vi "Instructor Write Client.vi"() -> ()   [LabVIEW 2017]
uses:
  <vilib>/OPCUA/controls/Write Status.ctl
  <vilib>/OPCUA/controls/NodeId.ctl
  <vilib>/OPCUA/client/Multiple Write Double Array.vi
  <vilib>/OPCUA/client/Multiple Write Bool Array.vi
  <vilib>/OPCUA/NI OPC UA Client.lvlib
panel:
  in  "Node Status 2":T1 items=["Good"=0, "Uncertain_InitialValue"=1083310080, "Uncertain_LastUsableValue"=1083179008, "Uncertain_SensorNotAccurate"=1083375616, "Uncertain_EngineeringUnitsExceeded"=1083441152, "Bad_NoCommunication"=2150694912, "Bad_NotReadable"=2151284736, "Bad_NotWritable"=2151350272, "Bad_OutOfRange"=2151415808, "Bad_WaitingForInitialData"=2150760448]
  in  "Time Stamp 2":timestamp
  in  "Node Status":T1 items=["Good"=0, "Uncertain_InitialValue"=1083310080, "Uncertain_LastUsableValue"=1083179008, "Uncertain_SensorNotAccurate"=1083375616, "Uncertain_EngineeringUnitsExceeded"=1083441152, "Bad_NoCommunication"=2150694912, "Bad_NotReadable"=2151284736, "Bad_NotWritable"=2151350272, "Bad_OutOfRange"=2151415808, "Bad_WaitingForInitialData"=2150760448]
  in  "Time Stamp":timestamp
  in  "Stop Broadcasting":bool
  in  "Time Stamp":timestamp
  in  "Node Status":T1 items=["Good"=0, "Uncertain_InitialValue"=1083310080, "Uncertain_LastUsableValue"=1083179008, "Uncertain_SensorNotAccurate"=1083375616, "Uncertain_EngineeringUnitsExceeded"=1083441152, "Bad_NoCommunication"=2150694912, "Bad_NotReadable"=2151284736, "Bad_NotWritable"=2151350272, "Bad_OutOfRange"=2151415808, "Bad_WaitingForInitialData"=2150760448]
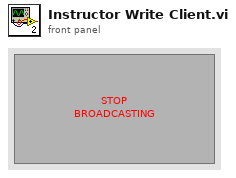
[diagram p1: front panel]
types:
  T1 = typedef "Write Status.ctl" = u32
  T2 = cluster{"message mode":enum16{"None", "Sign", "Sign and Encrypt"}, "security":enum16{"Basic256", "Basic128Rsa15"}}
  T3 = typedef "OPC UA Client Refnum.ctl" = refnum<k21>
  T4 = typedef "NodeId.ctl" = string
  T5 = cluster{"node ID":T4, "value":bool[], "timestamp (current time)":timestamp, "node status":T1}
  T6 = cluster{"node ID":T4, "value":dbl[], "timestamp (current time)":timestamp, "node status":T1}
  T7 = cluster{"node ID":T4, "value":dbl[], "timestamp (current time)":timestamp, "node status":T1}[]
  T8 = cluster{"node ID":T4, "value":bool[], "timestamp (current time)":timestamp, "node status":T1}[]
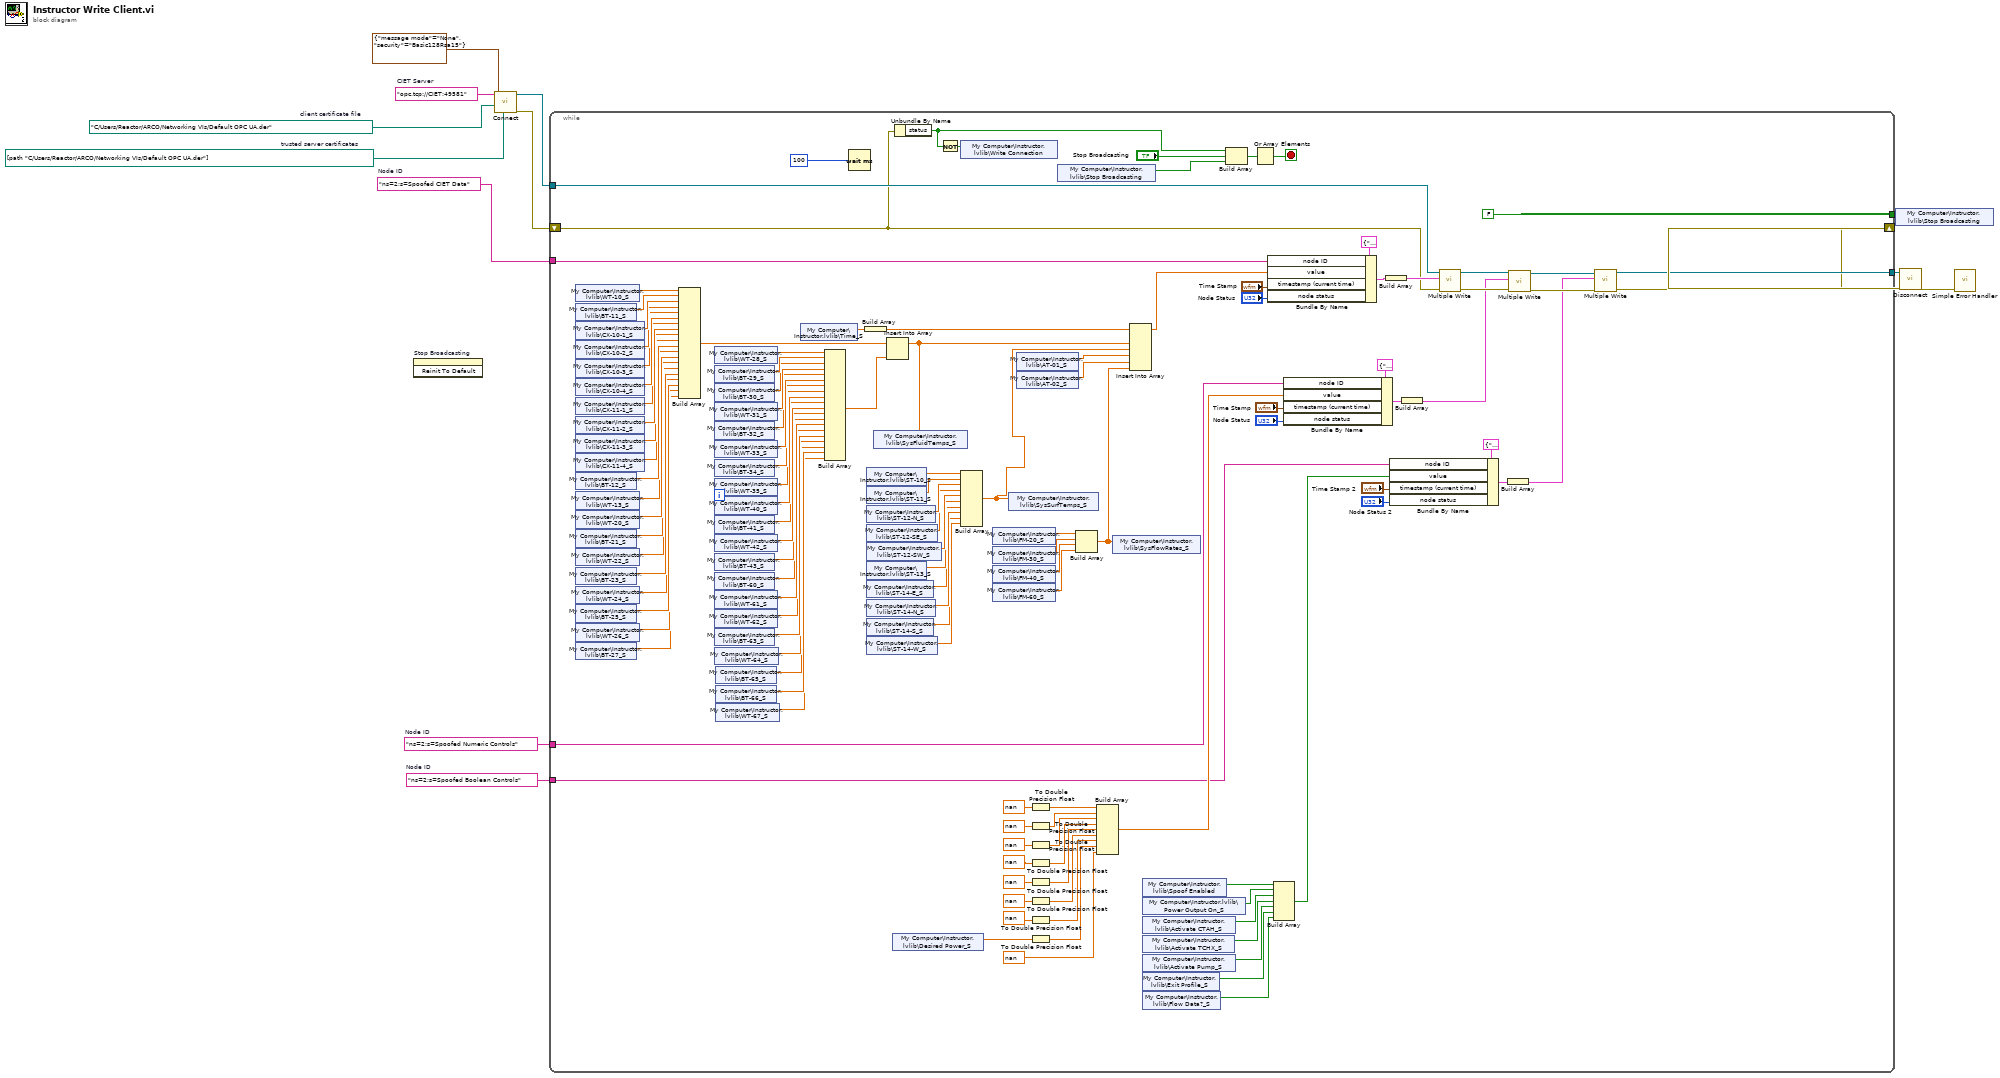
[diagram p0: block diagram]
diagram:
  w1 = "ns=2;s=Spoofed Boolean Controls"  # Node ID
  w3 = "ns=2;s=Spoofed Numeric Controls"  # Node ID
  w8 = path[] [path "C:/Users/Reactor/ARCO/Networking VIs/Default OPC UA.der"]  # trusted server certificates
  w9 = path "C:/Users/Reactor/ARCO/Networking VIs/Default OPC UA.der"  # client certificate file
  w10 = "ns=2;s=Spoofed CIET Data"  # Node ID
  w12 = "opc.tcp://CIET:49581"  # CIET Server
  n1 = invoke on="Stop Broadcasting" class="Bool (strict)" method="Reinit To Default"() -> ()  [unwired: 3 in, 3 out]
  n2 = call <vilib>:"Connect.vi"("trusted server certificates"=w8, "client certificate file"=w9, "security policy"=T2 {"message mode"=enum."None", "security"=enum."Basic128Rsa15"}, "server endpoint URL"=w12) -> ("error out"=w5:errorcluster, "OPC UA client refnum out"=w11:T3)  [unwired: 5 in, 1 out]
  n3 = while {
    tunnel: w10 -> [w136]
    tunnel: w11 -> [w135]
    tunnel: [FALSE] -> w6
    shift-right: [w24] -> w4
    shift-left: w5 -> [w58]
    tunnel: w3 -> [w52]
    tunnel: [w25] -> w2
    tunnel: w1 -> [w23]
    stop <- w64 stop-if-true
    n4 = shared-variable "My Computer\\Instructor.lvlib\\WT-10_S"() -> (w129:sgl)  [unwired: 1 in, 1 out]
    n5 = shared-variable "My Computer\\Instructor.lvlib\\BT-11_S"() -> (w128:sgl)  [unwired: 1 in, 1 out]
    n6 = shared-variable "My Computer\\Instructor.lvlib\\CX-10-1_S"() -> (w127:sgl)  [unwired: 1 in, 1 out]
    n7 = shared-variable "My Computer\\Instructor.lvlib\\CX-10-2_S"() -> (w126:sgl)  [unwired: 1 in, 1 out]
    n8 = shared-variable "My Computer\\Instructor.lvlib\\CX-10-3_S"() -> (w125:sgl)  [unwired: 1 in, 1 out]
    n9 = shared-variable "My Computer\\Instructor.lvlib\\CX-10-4_S"() -> (w124:sgl)  [unwired: 1 in, 1 out]
    n10 = shared-variable "My Computer\\Instructor.lvlib\\CX-11-1_S"() -> (w123:sgl)  [unwired: 1 in, 1 out]
    n11 = shared-variable "My Computer\\Instructor.lvlib\\CX-11-2_S"() -> (w122:sgl)  [unwired: 1 in, 1 out]
    n12 = shared-variable "My Computer\\Instructor.lvlib\\CX-11-3_S"() -> (w121:sgl)  [unwired: 1 in, 1 out]
    n13 = shared-variable "My Computer\\Instructor.lvlib\\CX-11-4_S"() -> (w120:sgl)  [unwired: 1 in, 1 out]
    n14 = shared-variable "My Computer\\Instructor.lvlib\\BT-12_S"() -> (w119:sgl)  [unwired: 1 in, 1 out]
    n15 = shared-variable "My Computer\\Instructor.lvlib\\WT-13_S"() -> (w118:sgl)  [unwired: 1 in, 1 out]
    n16 = shared-variable "My Computer\\Instructor.lvlib\\WT-20_S"() -> (w117:sgl)  [unwired: 1 in, 1 out]
    n17 = shared-variable "My Computer\\Instructor.lvlib\\BT-21_S"() -> (w116:sgl)  [unwired: 1 in, 1 out]
    n18 = shared-variable "My Computer\\Instructor.lvlib\\WT-22_S"() -> (w115:sgl)  [unwired: 1 in, 1 out]
    n19 = shared-variable "My Computer\\Instructor.lvlib\\BT-23_S"() -> (w114:sgl)  [unwired: 1 in, 1 out]
    n20 = shared-variable "My Computer\\Instructor.lvlib\\WT-24_S"() -> (w113:sgl)  [unwired: 1 in, 1 out]
    n21 = shared-variable "My Computer\\Instructor.lvlib\\BT-25_S"() -> (w112:sgl)  [unwired: 1 in, 1 out]
    n22 = shared-variable "My Computer\\Instructor.lvlib\\WT-26_S"() -> (w111:sgl)  [unwired: 1 in, 1 out]
    n23 = shared-variable "My Computer\\Instructor.lvlib\\BT-27_S"() -> (w110:sgl)  [unwired: 1 in, 1 out]
    n24 = Build Array(w129, w128, w127, w126, w125, w124, w123, w122, w121, w120, w119, w118, w117, w116, w115, w114, w113, w112, w111, w110) -> (w88:sgl[])
    n25 = shared-variable "My Computer\\Instructor.lvlib\\WT-28_S"() -> (w109:sgl)  [unwired: 1 in, 1 out]
    n26 = shared-variable "My Computer\\Instructor.lvlib\\BT-29_S"() -> (w108:sgl)  [unwired: 1 in, 1 out]
    n27 = shared-variable "My Computer\\Instructor.lvlib\\BT-30_S"() -> (w107:sgl)  [unwired: 1 in, 1 out]
    n28 = shared-variable "My Computer\\Instructor.lvlib\\WT-31_S"() -> (w106:sgl)  [unwired: 1 in, 1 out]
    n29 = shared-variable "My Computer\\Instructor.lvlib\\BT-32_S"() -> (w105:sgl)  [unwired: 1 in, 1 out]
    n30 = shared-variable "My Computer\\Instructor.lvlib\\WT-33_S"() -> (w104:sgl)  [unwired: 1 in, 1 out]
    n31 = shared-variable "My Computer\\Instructor.lvlib\\BT-34_S"() -> (w103:sgl)  [unwired: 1 in, 1 out]
    n32 = shared-variable "My Computer\\Instructor.lvlib\\WT-35_S"() -> (w102:sgl)  [unwired: 1 in, 1 out]
    n33 = shared-variable "My Computer\\Instructor.lvlib\\WT-40_S"() -> (w101:sgl)  [unwired: 1 in, 1 out]
    n34 = shared-variable "My Computer\\Instructor.lvlib\\BT-41_S"() -> (w100:sgl)  [unwired: 1 in, 1 out]
    n35 = shared-variable "My Computer\\Instructor.lvlib\\WT-42_S"() -> (w99:sgl)  [unwired: 1 in, 1 out]
    n36 = shared-variable "My Computer\\Instructor.lvlib\\BT-43_S"() -> (w98:sgl)  [unwired: 1 in, 1 out]
    n37 = shared-variable "My Computer\\Instructor.lvlib\\BT-60_S"() -> (w97:sgl)  [unwired: 1 in, 1 out]
    n38 = shared-variable "My Computer\\Instructor.lvlib\\WT-61_S"() -> (w96:sgl)  [unwired: 1 in, 1 out]
    n39 = shared-variable "My Computer\\Instructor.lvlib\\WT-62_S"() -> (w95:sgl)  [unwired: 1 in, 1 out]
    n40 = shared-variable "My Computer\\Instructor.lvlib\\BT-63_S"() -> (w94:sgl)  [unwired: 1 in, 1 out]
    n41 = shared-variable "My Computer\\Instructor.lvlib\\WT-64_S"() -> (w93:sgl)  [unwired: 1 in, 1 out]
    n42 = shared-variable "My Computer\\Instructor.lvlib\\BT-65_S"() -> (w92:sgl)  [unwired: 1 in, 1 out]
    n43 = shared-variable "My Computer\\Instructor.lvlib\\BT-66_S"() -> (w91:sgl)  [unwired: 1 in, 1 out]
    n44 = shared-variable "My Computer\\Instructor.lvlib\\WT-67_S"() -> (w90:sgl)  [unwired: 1 in, 1 out]
    n45 = shared-variable "My Computer\\Instructor.lvlib\\Time_S"() -> (w77:sgl)  [unwired: 1 in, 1 out]
    n46 = Build Array(w109, w108, w107, w106, w105, w104, w103, w102, w101, w100, w99, w98, w97, w96, w95, w94, w93, w92, w91, w90) -> (w89:sgl[])
    n47 = Wait (ms)(milliseconds to wait=u32 100) -> ()  [unwired: 1 out]
    n48 = Build Array(w77) -> (w68:sgl[])
    n49 = shared-variable "My Computer\\Instructor.lvlib\\ST-10_S"() -> (w87:sgl)  [unwired: 1 in, 1 out]
    n50 = shared-variable "My Computer\\Instructor.lvlib\\ST-11_S"() -> (w86:sgl)  [unwired: 1 in, 1 out]
    n51 = shared-variable "My Computer\\Instructor.lvlib\\ST-12-N_S"() -> (w85:sgl)  [unwired: 1 in, 1 out]
    n52 = shared-variable "My Computer\\Instructor.lvlib\\ST-12-SE_S"() -> (w84:sgl)  [unwired: 1 in, 1 out]
    n53 = shared-variable "My Computer\\Instructor.lvlib\\ST-12-SW_S"() -> (w83:sgl)  [unwired: 1 in, 1 out]
    n54 = shared-variable "My Computer\\Instructor.lvlib\\ST-13_S"() -> (w82:sgl)  [unwired: 1 in, 1 out]
    n55 = shared-variable "My Computer\\Instructor.lvlib\\ST-14-E_S"() -> (w81:sgl)  [unwired: 1 in, 1 out]
    n56 = shared-variable "My Computer\\Instructor.lvlib\\ST-14-N_S"() -> (w80:sgl)  [unwired: 1 in, 1 out]
    n57 = shared-variable "My Computer\\Instructor.lvlib\\ST-14-S_S"() -> (w79:sgl)  [unwired: 1 in, 1 out]
    n58 = shared-variable "My Computer\\Instructor.lvlib\\ST-14-W_S"() -> (w78:sgl)  [unwired: 1 in, 1 out]
    n59 = Insert Into Array(array=w88, new element=w89) -> (w76:sgl[])  [unwired: 1 in]
    n60 = shared-variable "My Computer\\Instructor.lvlib\\SysFluidTemps_S"(w76) -> ()  [unwired: 1 in, 1 out]
    n61 = shared-variable "My Computer\\Instructor.lvlib\\Desired Power_S"() -> (w45:sgl)  [unwired: 1 in, 1 out]
    n62 = Unbundle By Name(w58) -> ("status"=w60:bool)
    n63 = Not(x=w60) -> (.not. x?=w59:bool)
    n64 = shared-variable "My Computer\\Instructor.lvlib\\Write Connection"(w59) -> ()  [unwired: 1 in, 1 out]
    n65 = Build Array(w87, w86, w85, w84, w83, w82, w81, w80, w79, w78) -> (w67:sgl[])
    n66 = shared-variable "My Computer\\Instructor.lvlib\\FM-20_S"() -> (w73:sgl)  [unwired: 1 in, 1 out]
    n67 = shared-variable "My Computer\\Instructor.lvlib\\FM-30_S"() -> (w72:sgl)  [unwired: 1 in, 1 out]
    n68 = shared-variable "My Computer\\Instructor.lvlib\\FM-40_S"() -> (w71:sgl)  [unwired: 1 in, 1 out]
    n69 = shared-variable "My Computer\\Instructor.lvlib\\FM-60_S"() -> (w70:sgl)  [unwired: 1 in, 1 out]
    n70 = shared-variable "My Computer\\Instructor.lvlib\\SysSurfTemps_S"(w67) -> ()  [unwired: 1 in, 1 out]
    n71 = shared-variable "My Computer\\Instructor.lvlib\\AT-01_S"() -> (w75:sgl)  [unwired: 1 in, 1 out]
    n72 = shared-variable "My Computer\\Instructor.lvlib\\AT-02_S"() -> (w74:sgl)  [unwired: 1 in, 1 out]
    n73 = To Double Precision Float(number=nan) -> (double precision float=w49:dbl)
    n74 = To Double Precision Float(number=nan) -> (double precision float=w48:dbl)
    n75 = To Double Precision Float(number=nan) -> (double precision float=w47:dbl)
    n76 = To Double Precision Float(number=nan) -> (double precision float=w46:dbl)
    n77 = To Double Precision Float(number=nan) -> (double precision float=w44:dbl)
    n78 = To Double Precision Float(number=nan) -> (double precision float=w43:dbl)
    n79 = To Double Precision Float(number=nan) -> (double precision float=w42:dbl)
    n80 = To Double Precision Float(number=w45) -> (double precision float=w41:dbl)
    n81 = shared-variable "My Computer\\Instructor.lvlib\\Stop Broadcasting"() -> (w62:bool)  [unwired: 1 in, 1 out]
    n82 = Build Array(w73, w72, w71, w70) -> (w69:sgl[])
    n83 = Build Array(w49, w48, w47, w46, w44, w43, w42, w41, nan ("number")) -> (w40:dbl[])
    n84 = shared-variable "My Computer\\Instructor.lvlib\\SysFlowRates_S"(w69) -> ()  [unwired: 1 in, 1 out]
    n85 = Insert Into Array(array=w68, new element #1=w76, new element #2=w67, new element #3=w75, new element #4=w74, new element #5=w69) -> (w66:sgl[])  [unwired: 1 in]
    n86 = shared-variable "My Computer\\Instructor.lvlib\\Spoof Enabled"() -> (w21:bool)  [unwired: 1 in, 1 out]
    n87 = shared-variable "My Computer\\Instructor.lvlib\\Power Output On_S"() -> (w20:bool)  [unwired: 1 in, 1 out]
    n88 = shared-variable "My Computer\\Instructor.lvlib\\Activate CTAH_S"() -> (w19:bool)  [unwired: 1 in, 1 out]
    n89 = shared-variable "My Computer\\Instructor.lvlib\\Activate TCHX_S"() -> (w18:bool)  [unwired: 1 in, 1 out]
    n90 = shared-variable "My Computer\\Instructor.lvlib\\Activate Pump_S"() -> (w17:bool)  [unwired: 1 in, 1 out]
    n91 = shared-variable "My Computer\\Instructor.lvlib\\Exit Profile_S"() -> (w16:bool)  [unwired: 1 in, 1 out]
    n92 = shared-variable "My Computer\\Instructor.lvlib\\Flow Data?_S"() -> (w15:bool)  [unwired: 1 in, 1 out]
    n93 = Build Array(w60, "Stop Broadcasting", w62) -> (w63:bool[])
    n94 = Or Array Elements(Boolean array=w63) -> (logical OR=w64:bool)
    n95 = Bundle By Name(cluster=T6 {"node ID"="", "value"=[], "timestamp (current time)"=timestamp(0 s since 1904-01-01), "node status"=0} ("request"), "node ID"=w136, "value"=w66, "timestamp (current time)"="Time Stamp", "node status"="Node Status") -> (w131:T6)
    n96 = Build Array(w21, w20, w19, w18, w17, w16, w15) -> (w22:bool[])
    n97 = Bundle By Name(cluster=T6 {"node ID"="", "value"=[], "timestamp (current time)"=timestamp(0 s since 1904-01-01), "node status"=0} ("request"), "node ID"=w52, "value"=w40, "timestamp (current time)"="Time Stamp", "node status"="Node Status") -> (w55:T6)
    n98 = Build Array(w131) -> (w130:T7)
    n99 = Bundle By Name(cluster=T5 {"node ID"="", "value"=[], "timestamp (current time)"=timestamp(0 s since 1904-01-01), "node status"=0} ("request"), "node ID"=w23, "value"=w22, "timestamp (current time)"="Time Stamp 2", "node status"="Node Status 2") -> (w31:T5)
    n100 = Build Array(w55) -> (w54:T7)
    n101 = call-poly <vilib>:"Multiple Write.vi"("error in (no error)"=w58, "requests"=w130, "OPC UA client refnum in"=w135) -> ("error out"=w56:errorcluster, "OPC UA client refnum out"=w57:T3)  [unwired: 5 in, 2 out]
    n102 = Build Array(w31) -> (w14:T8)
    n103 = call-poly <vilib>:"Multiple Write.vi"("error in (no error)"=w56, "requests"=w54, "OPC UA client refnum in"=w57) -> ("error out"=w26:errorcluster, "OPC UA client refnum out"=w27:T3)  [unwired: 5 in, 2 out]
    n104 = call-poly <vilib>:"Multiple Write.vi"("error in (no error)"=w26, "requests"=w14, "OPC UA client refnum in"=w27) -> ("error out"=w24:errorcluster, "OPC UA client refnum out"=w25:T3)  [unwired: 5 in, 2 out]
  }
  n105 = shared-variable "My Computer\\Instructor.lvlib\\Stop Broadcasting"(w6) -> ()  [unwired: 1 in, 1 out]
  n106 = call <vilib>:"Disconnect.vi"("error in (no error)"=w4, "OPC UA client refnum in"=w2) -> ("error out"=w13:errorcluster)  [unwired: 9 in]
  n107 = call <vilib>:"Simple Error Handler.vi"("error in (no error)"=w13) -> ()  [unwired: 4 in, 5 out]
